vi "Initialize.vi"(8 "error in (no error)":errorcluster) -> (0 "error out":errorcluster, 3 "Idle out":refnum<class "Idle.lvclass">)   [LabVIEW 2011, in "Idle.lvclass"]
uses:
  Idle.lvclass
  2 Globals/2 Global.vi
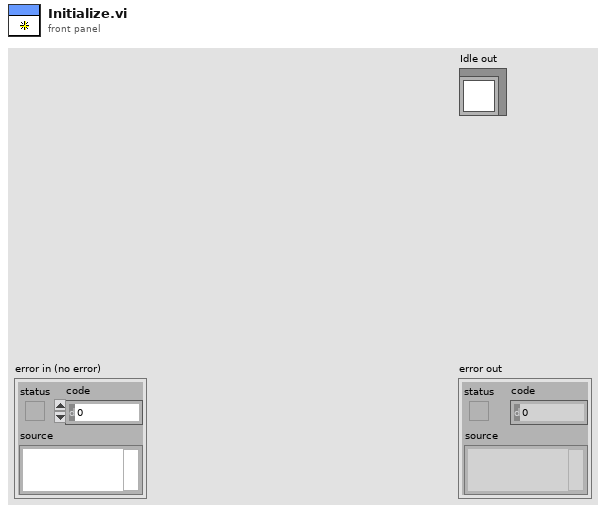
[diagram p1: front panel]
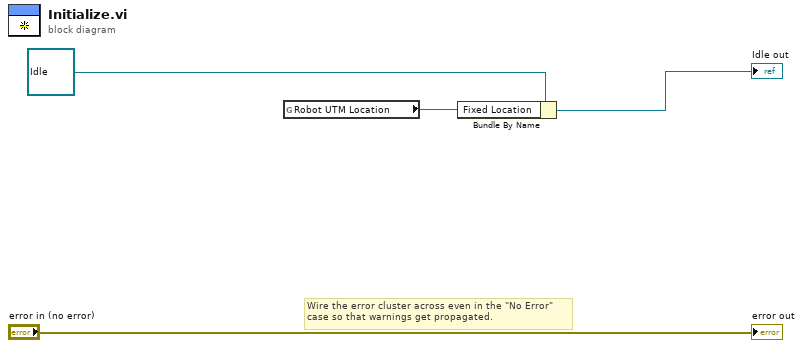
[diagram p0: block diagram]
diagram:
  # "Wire the error cluster across even in the \"No Error\"\ncase so that warnings get propagated."
  n1 = global read "2 Global.vi" "Robot UTM Location"() -> (w1:refnum<class "UTM_Location.lvclass">)
  n2 = Bundle By Name(cluster=refnum<class "Idle.lvclass"> refnum ("Idle out"), "Fixed Location"=w1) -> (→"Idle out":refnum<class "Idle.lvclass">)
  "error out" <- "error in (no error)"
